vi "analizzatore di spettro.vi"() -> ()   [LabVIEW 2018]
uses:
  <vilib>/Analysis/4window.llb/windowTd.ctl
  <vilib>/measure/maspectr.llb/FFT Spectrum (Mag-Phase) for 1 Chan.vi
  <vilib>/measure/NI_MAPro.lvlib
  <vilib>/measure/NI_MABase.lvlib
  <vilib>/Analysis/NI_AALPro.lvlib
panel:
  in  "df":dbl=0.02 min=0.0 step=0.1
  in  "Tab Control":enum32{"start/stop", "centro & span"}(tab)
  in  "f start":dbl min=0.0 step=1.0
  in  "f stop":dbl=1.0 min=0.0 step=1.0
  in  "span":dbl=50.0 min=0.0 step=1.0 format="%0.2p"
  in  "Center freq":dbl=500.0 min=0.0 step=1.0 format="%0.2p"
  out "fc":dbl=5.12 min=0.0 step=1.0
  in  "tones":T1(array[cluster])=[{"frequency"=0.2, "amplitude"=1.0, "phase"=0.0}, {"frequency"=0.0, "amplitude"=1.0, "phase"=0.0}] {"phase" format="%.2p"; "amplitude" min=0.0 step=0.1 format="%0.2p"; "frequency" min=0.0 step=0.1 format="%0.2p"}
  in  "window":T2 items=["Rectangle"=0, "Hanning"=1, "Hamming"=2, "Blackman-Harris"=3, "Exact Blackman"=4, "Blackman"=5, "Flat Top"=6, "4 Term B-Harris "=7, "7 Term B-Harris"=8, "Low Sidelobe"=9, "Blackman Nuttall"=11, "Triangle"=30, "Bartlett-Hanning"=31, "Bohman"=32, "Parzen"=33, "Welch"=34, "Kaiser"=60, "Dolph-Chebyshev"=61, "Gaussian"=62]
  in  "scala y":string(combo)="linear"
  out "N":dbl=256.0
  in  "frequency":string(combo)="start/stop"
  in  "stop":bool
  out "spettro di frequenza":cluster{"f0":dbl, "df":dbl, "magnitude":dbl[]}(graph)={"f0"=0.0, "df"=0.02, "magnitude"=[1.4094628242311558e-17, 2.5189114516830814e-17, 2.482470956464378e-17, 4.0543142819399115e-17, 5.753683036667772e-17, 7.570583572611535e-17, 9.22998684659014e-17, 1.4491179310372326e-16, 2.397697909587037e-16, 4.812661237675266e-16, 0.7071067811865475, 5.395239259726897e-16, 2.7224501157389184e-16, 2.1001466219670863e-16, 1.4158184580597952e-16, 1.3018533869519184e-16, 1.0864382804365327e-16, 9.113489473109625e-17, 8.207983566926925e-17, 7.923626489277622e-17, 7.671804831327016e-17, 6.199791554346821e-17, 4.7167467542078855e-17, 5.617376054563885e-17, 5.3658455809746177e-17, 5.195017368978431e-17, 3.531909035721208e-17, 4.699548347662591e-17, 4.339485017759543e-17, 3.851803801652829e-17, 4.372447415461251e-17, 3.6548989264455153e-17, 3.6080628390017695e-17, 3.8197048672624046e-17, 3.18863412206376e-17, 3.3642842194562033e-17, 3.172524419258872e-17, 3.0007170319387345e-17, 2.2289547913012113e-17, 2.7411058634115244e-17, 2.638449422788657e-17, 2.7552031160430024e-17, 1.717064858435908e-17, 2.73928502892226e-17, 2.800403151862976e-17, 2.4510971099143843e-17, 2.8447996627257557e-17, 2.2100825283809918e-17, 2.6208910673901762e-17, 2.628786490417723e-17, 1.9695368052948897e-17, 2.4387793971616475e-17, 2.4343430619485647e-17, 2.1699250755011182e-17, 2.955618140848143e-17, 1.9853360117018844e-17, 2.06466734286645e-17, 2.1200672246822325e-17, 2.8187130320288566e-17, 2.023590647606456e-17, 2.1512055175344776e-17, 1.9551116121522484e-17, 2.6193874402891572e-17, 1.8398790125077495e-17, 1.6933002747669192e-17, 1.705987022744675e-17, 3.362711372912798e-17, 2.011507143099152e-17, 1.9053117299297302e-17, 1.70970919618973e-17, 1.544354895818233e-17, 1.7530236435545658e-17, 1.5220147687889447e-17, 1.5082312706864403e-17, 4.911174471654556e-17, 1.64687000139771e-17, 1.7480481475366494e-17, 1.8394861479944826e-17, 2.6010583324778808e-17, 1.6239749490531637e-17, 1.2851759664954917e-17, 1.5989165412078154e-17, 1.3897736700544337e-17, 1.5865450627772635e-17, 1.563517955057551e-17, 1.6442590950814595e-17, 5.555810570685253e-17, 1.2154544198556336e-17, 1.3947132870084605e-17, 1.6561389077569845e-17, 2.5385580014731444e-18, 1.6526094340995465e-17, 1.5172862294345442e-17, 1.5739797060808104e-17, 1.9055558450171938e-17, 1.1937905276358459e-17, 1.67143416310522e-17, 1.4285437659495856e-17, 9.428282707088322e-18, 1.36826924939613e-17, 1.890519162921609e-17, 1.4081924858990424e-17, 2.1544114297939715e-17, 1.5201915079073694e-17, 1.464510092641146e-17, 1.6676929076761436e-17, 1.9656864207024374e-17, 1.548915973898466e-17, 1.505028564622725e-17, 1.4992015068365773e-17, 2.6287309937020293e-17, 1.363706830187405e-17, 2.399600624434084e-17, 2.9188704402869776e-17, 1.8930297277926638e-17, 7.956894134308568e-18, 2.4751482160058225e-17, 4.286083785383035e-17, 9.66700114382585e-17, 4.3715482858857884e-17, 5.1281456117142735e-17, 1.8928494837527428e-17, 1.2737850524486656e-17, 6.813489040289468e-18, 4.510117189775994e-18, 5.1614386512670374e-18, 9.954211254034289e-18, 7.872658996215512e-18]}
  # "SEGNALE IN INGRESSO"
  # "SPETTRO DI FREQUENZA"
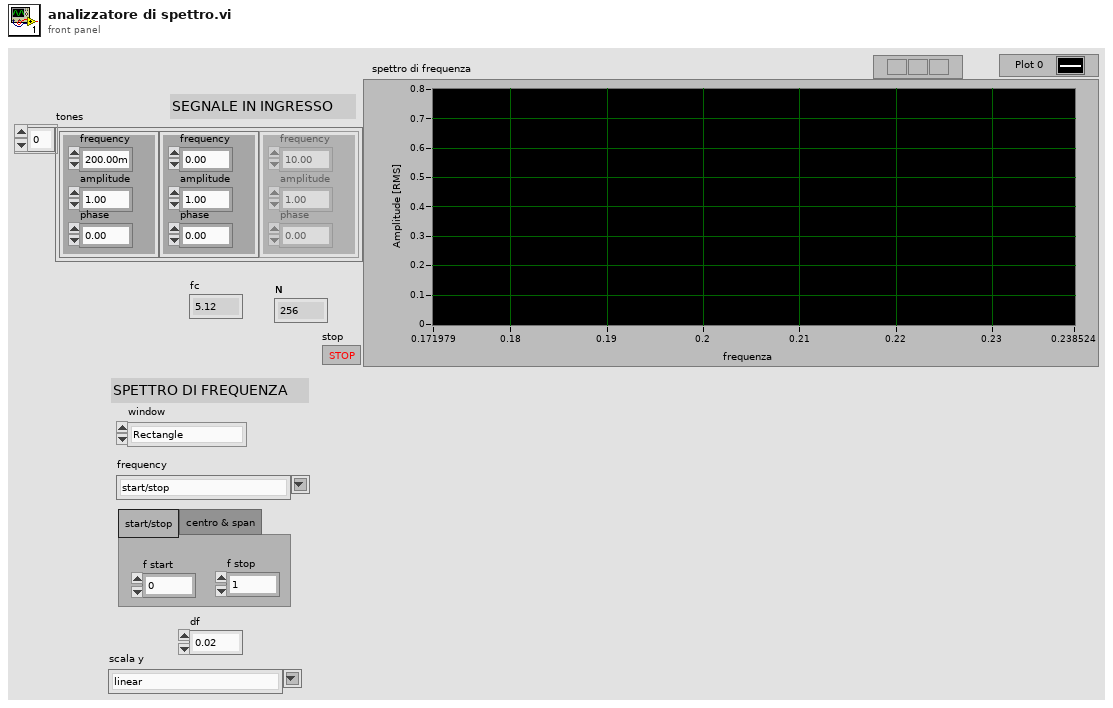
[diagram p1: front panel]
types:
  T1 = cluster{"frequency":dbl, "amplitude":dbl, "phase":dbl}[]
  T2 = typedef "NI_AALPro.lvlib/windowTd.ctl" = u32
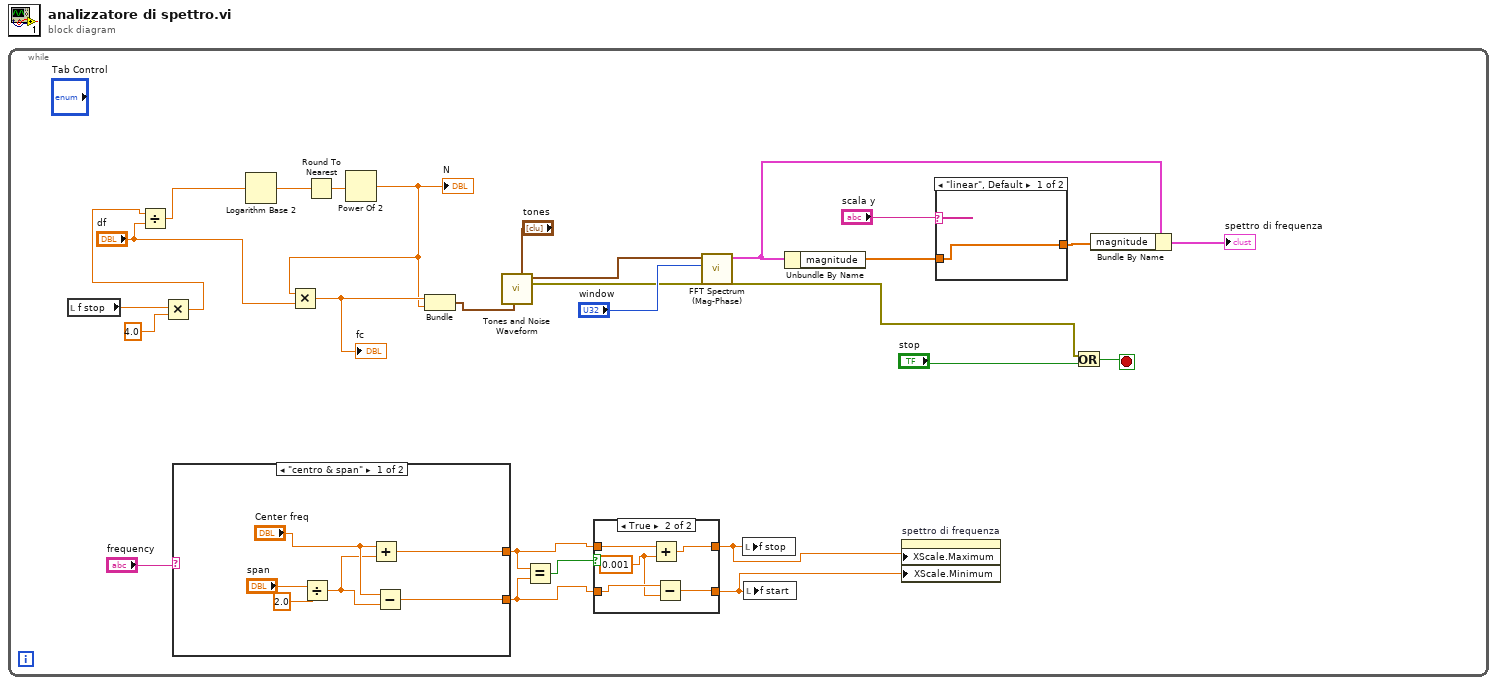
[diagram p0: block diagram]
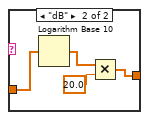
[diagram p3: hidden frame]
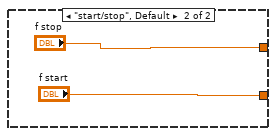
[diagram p4: hidden frame]
diagram:
  n1 = while {
    stop <- w27 stop-if-true
    n2 = local read "f stop"() -> (w9:dbl)
    n3 = Multiply(x=w9, y=4.0) -> (x*y=w4:dbl)
    n4 = Divide(x=w4, y="df") -> (x/y=w8:dbl)
    n5 = case shown="\"centro & span\"" "frequency" {
      tunnel: [w42 "f stop"] -> w22
      tunnel: [w41 "f start"] -> w23
      frame "centro & span" {
        n6 = Divide(x="span", y=2.0) -> (x/y=w43:dbl)
        n7 = Add(x="Center freq", y=w43) -> (x+y=w42:dbl)
        n8 = Subtract(x="Center freq", y=w43) -> (x-y=w41:dbl)
      }
      frame "start/stop", Default {
      }
    }
    n9 = Logarithm Base 2(1:w8) -> (0:w6:dbl)
    n10 = Round To Nearest(number=w6) -> (nearest integer value=w5:dbl)
    n11 = Power Of 2(x=w5) -> (2^x=w1:dbl)
    "N" <- w1
    n12 = Multiply(x=w1, y="df") -> (x*y=w2:dbl)
    "fc" <- w2
    n13 = Bundle(w2, w1) -> (w17:cluster{dbl, dbl})  [unwired: 1 in]
    n14 = call <vilib>:"Tones and Noise Waveform.vi"("sampling info"=w17, "tones"="tones") -> ("error out"=w18:errorcluster, "signal out"=w16:waveform(dbl))  [unwired: 8 in]
    n15 = Equal?(x=w22, y=w23) -> (x = y?=w24:bool)
    n16 = case shown="True" w24 {
      tunnel: w23 -> [w29 w34]
      tunnel: w22 -> [w30 w35]
      tunnel: [w30 w31] -> w11
      tunnel: [w29 w32] -> w10
      frame False {
      }
      frame True {
        w33 = 0.001 ("y")
        n17 = Add(x=w35, y=w33) -> (x+y=w31:dbl)
        n18 = Subtract(x=w34, y=w33) -> (x-y=w32:dbl)
      }
    }
    n19 = call-poly <vilib>:"FFT Spectrum (Mag-Phase).vi"("error in (no error)"=w18, "window"="window", "time signal"=w16) -> ("error out"=w19:errorcluster, "magnitude"=w15:cluster{"f0":dbl, "df":dbl, "magnitude":dbl[]})  [unwired: 4 in, 3 out]
    n20 = local write "f stop"(w11) -> ()
    n21 = local write "f start"(w10) -> ()
    n22 = Unbundle By Name(w15) -> ("magnitude"=w14:dbl[])
    n23 = property on="spettro di frequenza" class="WFGraph (strict)"("XScale.Maximum"=w11, "XScale.Minimum"=w10) -> ()  [unwired: 2 in, 2 out]
    n24 = case shown="\"linear\", Default" "scala y" {
      tunnel: [w36 w38] -> w13
      tunnel: w14 -> [w36 w37]
      frame "linear", Default {
      }
      frame "dB" {
        n25 = Logarithm Base 10(1:w37) -> (0:w40:dbl[])
        n26 = Multiply(x=w40, y=20.0) -> (x*y=w38:dbl[])
      }
    }
    n27 = Or(x=w19, y="stop") -> (x .or. y?=w27:bool)
    n28 = Bundle By Name(cluster=w15, "magnitude"=w13) -> (→"spettro di frequenza":cluster{"f0":dbl, "df":dbl, "magnitude":dbl[]})
  }
